vi "CANframeSelect.vi"(10 "CANID":string, 11 "重构的Data数组输入":u32[][](array[numeric])) -> (2 "筛选的报文数组":u32[][](array[numeric]), 3 "报文数量":i32)   [LabVIEW 2015]
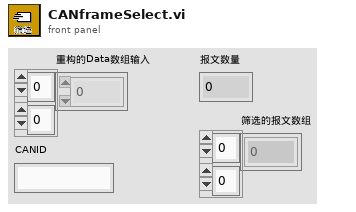
[diagram p1: front panel]
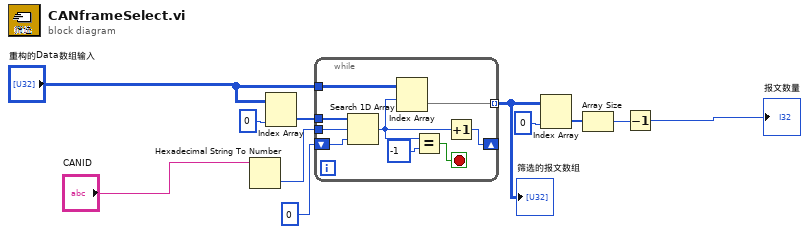
[diagram p0: block diagram]
diagram:
  n1 = Hexadecimal String To Number(string="CANID") -> (number=w5:u32)  [unwired: 2 in, 1 out]
  n2 = Index Array(array="重构的Data数组输入", index (col)=0 ("禁用的索引 (列)")) -> (element=w3:u32[])  [unwired: 1 in]
  n3 = while {
    tunnel: w3 -> [w20]
    tunnel: w5 -> [w18]
    tunnel: "重构的Data数组输入" -> [w17]
    tunnel: [w16] -> w10 mode=indexing
    shift-right: [w13] -> _
    shift-left: 0 -> [w19]
    stop <- w15 stop-if-true
    n4 = Search 1D Array(1D array=w20, element=w18, start index (0)=w19) -> (index of element=w12:i32)
    n5 = Index Array(array=w17, index (row)=w12) -> (element=w16:u32[])  [unwired: 1 in]
    n6 = Equal?(x=w12, y=-1) -> (x = y?=w15:bool)
    n7 = Increment(x=w12) -> (x+1=w13:i32)
  }
  "筛选的报文数组" <- w10
  n8 = Index Array(array=w10, index (col)=0 ("禁用的索引 (列)")) -> (element=w8:u32[])  [unwired: 1 in]
  n9 = Array Size(array=w8) -> (size(s)=w6:i32)
  n10 = Decrement(x=w6) -> (x-1=→"报文数量":i32)
